vi "Format LV Error as JSON Data.vi"(10 "error in":errorcluster) -> (0 "error out":errorcluster, 2 "Error Data Out":variant)   [LabVIEW 2015, in "JSONRPC Server.lvclass"]
doc: "This converts a LabVIEW Error to a JSON Tree for use with \"Add Response - Server Error\"."
uses:
  JSONRPC Server.lvclass
  <vilib>/rajsite/i3-json/JSON Generation/Create Value Files/Create Value - Object.vi
  <vilib>/rajsite/i3-json/JSON Generation/Add Object Parameter Files/Add Object Parameter - Numeric.vi
  <vilib>/rajsite/i3-json/JSON Generation/Add Object Parameter Files/Add Object Parameter - String.vi
  <vilib>/rajsite/i3-json/i3-json.lvlib
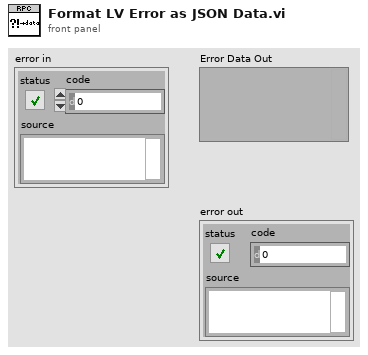
[diagram p1: front panel]
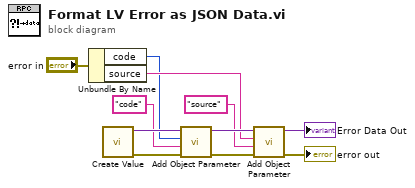
[diagram p0: block diagram]
diagram:
  n1 = Unbundle By Name("error in") -> ("code"=w2:i32, "source"=w3:string)
  n2 = call-poly <vilib>:"Create Value.vi"() -> ("error out"=w9:errorcluster, "JSON Tree"=w6:variant)  [unwired: 10 in]
  n3 = call-poly <vilib>:"Add Object Parameter.vi"("error in (no error)"=w9, "Name"="code", "Numeric"=w2, "JSON Tree in (JSON Object)"=w6) -> ("error out"=w10:errorcluster, "JSON Tree out (JSON Object)"=w7:variant)  [unwired: 6 in]
  n4 = call-poly <vilib>:"Add Object Parameter.vi"("error in (no error)"=w10, "Name"="source", "String"=w3, "JSON Tree in (JSON Object)"=w7) -> ("error out"=→"error out":errorcluster, "JSON Tree out (JSON Object)"=→"Error Data Out":variant)  [unwired: 6 in]
